vi "Ramsete_Execute_Ext_Odom.vi"(4 "Enabled":bool=TRUE, 6 "Reset":bool, 7 "RAMSETE_EXE_TUNING SI":T4={"B"=2.0, "Zeta"=0.7, "X Tolerance M"=2.0, "Y Tolerance M"=0.7, "Heading Tolerance RAD"=0.7, "Track Width M"=2.0, "Max Speed M/S"=2.0} {"Max Speed M/S" format="%13.4f"; "Track Width M" format="%13.4f"; "Heading Tolerance RAD" format="%13.4f"; "Y Tolerance M" format="%13.4f"; "X Tolerance M" format="%13.4f"; "Zeta" format="%13.4f"; "B" format="%13.4f"}, 9 "Current Pose SI":T1 {"ROTATION"."SIN" format="%13.4f"; "ROTATION"."COS" format="%13.4f"; "ROTATION"."VALUE" format="%13.4f"; "TRANSLATION"."Y" format="%14.3f"; "TRANSLATION"."X" format="%14.3f"}, 11 "TRAJ_STATE SI":T6 {"POSE"."ROTATION"."SIN" format="%13.4f"; "POSE"."ROTATION"."COS" format="%13.4f"; "POSE"."ROTATION"."VALUE" format="%13.4f"; "POSE"."TRANSLATION"."Y" format="%14.3f"; "POSE"."TRANSLATION"."X" format="%14.3f"}) -> (1 "AtReference":bool, 2 "Right Speed Dmd M/S":dbl, 3 "Left Speed Dmd M/S":dbl, 5 "outRAMSETE":T5={"B"=2.0, "Zeta"=0.7, "poseTolerance"={"TRANSLATION"={"X"=0.0, "Y"=0.0}, "ROTATION"={"VALUE"=0.0, "COS"=1.0, "SIN"=0.0}}, "poseError"={"TRANSLATION"={"X"=0.0, "Y"=0.0}, "ROTATION"={"VALUE"=0.0, "COS"=1.0, "SIN"=0.0}}, "Enabled"=TRUE} {"poseError"."ROTATION"."SIN" format="%13.4f"; "poseError"."ROTATION"."COS" format="%13.4f"; "poseError"."ROTATION"."VALUE" format="%13.4f"; "poseError"."TRANSLATION"."Y" format="%14.3f"; "poseError"."TRANSLATION"."X" format="%14.3f"; "poseTolerance"."ROTATION"."SIN" format="%13.4f"; "poseTolerance"."ROTATION"."COS" format="%13.4f"; "poseTolerance"."ROTATION"."VALUE" format="%13.4f"; "poseTolerance"."TRANSLATION"."Y" format="%14.3f"; "poseTolerance"."TRANSLATION"."X" format="%14.3f"; "Zeta" format="%12.3f"; "B" format="%12.3f"})   [LabVIEW 2019, in "Trajectory_Library.lvlib"]
doc: "Convienience function to create and calculate the ramsete control, returning normalized desired left and right speed setpoints \n\n\nParameters: \n - Ramsete EXE Tuning -- Packed data cluster containing the ramsete tuning parameters and Differntial Drive kinematics information. (SI Units)\n - TrajState - Desired trajectory state (SI Units)\n - Current Pose -- Current Pose2d robot location. (SI Units)\n - Reset -- Resets the Ramsete data structure.\n - Enabled -- When enabled uses the ramsete closed loop control to drive the left and right speed demand outputs. When disabled the trajectory data is directly converted to left and right speed demands.\n\n\nReturns:\n - Left Speed Dmd -- Left Speed demand (Meters/Second)\n - Right Speed Dmd -- Right Speed demand (Meters/Second)\n - Out Ramsete -- Updated Ramsete data structure (SI Units)\n - At Reference -- Set to TRUE when the current robot pose is withing the specified tolerance of the desired POSE from the trajectory state input."
uses:
  Trajectory_Library.lvlib
  TypeDef/TRAJ_STATE.ctl
  TypeDef/POSE2D.ctl
  TypeDef/TRANSLATION2D.ctl
  TypeDef/ROTATION2D.ctl
  TypeDef/RAMSETE.ctl
  TypeDef/RAMSETE_EXE_TUNING.ctl
  Rotation2d_CreateAngle.vi
  Translation2d_Create.vi
  <vilib>/Rock Robotics/SystemInterfaces/NetworkCommunication/NetComm_UsageReport_report.vi
  Globals/Util_LibraryGlobals.vi
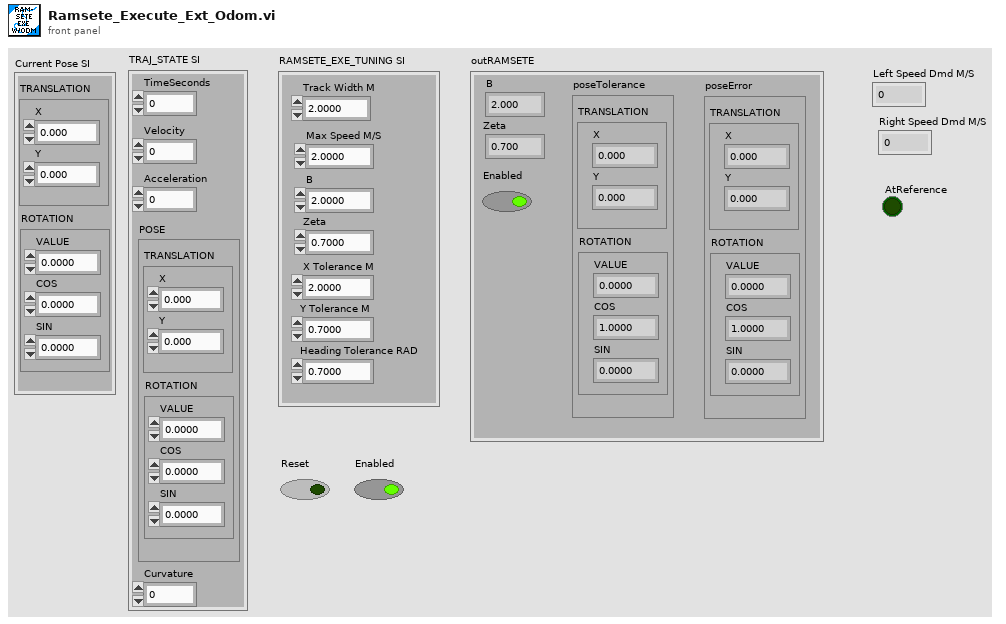
[diagram p1: front panel]
types:
  T1 = typedef "Trajectory_Library.lvlib/POSE2D.ctl" = cluster{"TRANSLATION":T2, "ROTATION":T3}
  T2 = typedef "Trajectory_Library.lvlib/TRANSLATION2D.ctl" = cluster{"X":dbl, "Y":dbl}
  T3 = typedef "Trajectory_Library.lvlib/ROTATION2D.ctl" = cluster{"VALUE":dbl, "COS":dbl, "SIN":dbl}
  T4 = typedef "Trajectory_Library.lvlib/RAMSETE_EXE_TUNING.ctl" = cluster{"B":dbl, "Zeta":dbl, "X Tolerance M":dbl, "Y Tolerance M":dbl, "Heading Tolerance RAD":dbl, "Track Width M":dbl, "Max Speed M/S":dbl}
  T5 = typedef "Trajectory_Library.lvlib/RAMSETE.ctl" = cluster{"B":dbl, "Zeta":dbl, "poseTolerance":T1, "poseError":T1, "Enabled":bool}
  T6 = typedef "Trajectory_Library.lvlib/TRAJ_STATE.ctl" = cluster{"TimeSeconds":dbl, "Velocity":dbl, "Acceleration":dbl, "POSE":T1, "Curvature":dbl}
  T7 = typedef "Trajectory_Library.lvlib/DIFF_DRIVE_KINEMATICS.ctl" = cluster{"TrackWidth_Meters":dbl}
  T8 = typedef "Trajectory_Library.lvlib/CHASSIS_SPEEDS.ctl" = cluster{"vX":dbl, "vY":dbl, "vOmega":dbl}
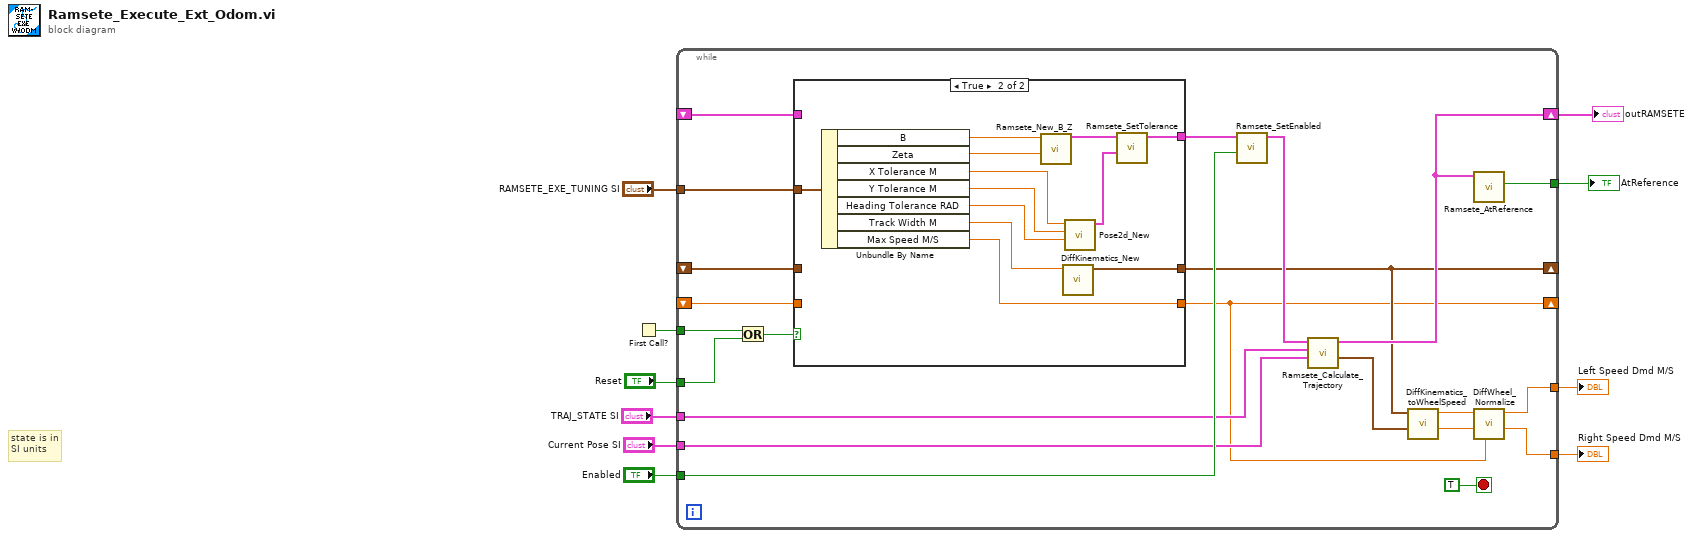
[diagram p0: block diagram]
diagram:
  # "state is in\nSI units"
  n1 = First Call?() -> (First Call?: T/F=w2:bool)
  n2 = while {
    tunnel: "RAMSETE_EXE_TUNING SI" -> [w13]
    tunnel: "TRAJ_STATE SI" -> [w17]
    tunnel: [w30] -> w6
    tunnel: [w29] -> w5
    tunnel: "Enabled" -> [w27]
    tunnel: "Reset" -> [w32]
    tunnel: [w21] -> w4
    tunnel: w2 -> [w26]
    shift-right: [w20] -> w8
    shift-left: _ -> [w25]
    tunnel: "Current Pose SI" -> [w16]
    shift-right: [w15] -> _
    shift-left: _ -> [w14]
    shift-right: [w12] -> _
    shift-left: _ -> [w11]
    stop <- TRUE stop-if-true
    n3 = Or(x=w26, y=w32) -> (x .or. y?=w31:bool)
    n4 = case shown="True" w31 {
      tunnel: [w35 w45] -> w28
      tunnel: w25 -> [w35 _]
      tunnel: [w34 w44] -> w15
      tunnel: w14 -> [w34 _]
      tunnel: [w33 w36] -> w12
      tunnel: w13 -> [_ w43]
      tunnel: w11 -> [w33 _]
      frame False {
      }
      frame True {
        n5 = Unbundle By Name(w43) -> ("B"=w42:dbl, "Zeta"=w41:dbl, "X Tolerance M"=w40:dbl, "Y Tolerance M"=w39:dbl, "Heading Tolerance RAD"=w38:dbl, "Track Width M"=w37:dbl, "Max Speed M/S"=w36:dbl)
        n6 = call "Ramsete_New_B_Z.vi"("Zeta"=w41, "B"=w42) -> ("outRAMSETE"=w47:T5)  [unwired: 9 in]
        n7 = call "DiffKinematics_New.vi"("TrackWidth_Meters"=w37) -> ("DIFF_DRIVE_KINEMATICS"=w44:T7)  [unwired: 10 in]
        n8 = call "Pose2d_New.vi"("Heading"=w38, "Y"=w39, "X"=w40) -> ("out POSe"=w46:T1)  [unwired: 8 in]
        n9 = call "Ramsete_SetTolerance.vi"("tolerancePose"=w46, "inRAMSETE"=w47) -> ("outRAMSETE"=w45:T5)  [unwired: 9 in]
      }
    }
    n10 = call "Ramsete_SetEnabled.vi"("Enabled"=w27, "inRAMSETE"=w28) -> ("outRAMSETE"=w22:T5)  [unwired: 9 in]
    n11 = call "Ramsete_Calculate_Trajectory.vi"("CurrentPOSE"=w16, "TRAJ_STATE"=w17, "inRAMSETE"=w22) -> ("CHASSIS Speeds"=w23:T8, "outRAMSETE"=w20:T5)  [unwired: 7 in]
    n12 = call "DiffKinematics_toWheelSpeed.vi"("CHASSIS Speed"=w23, "DIFF_DRIVE_KINEMATICS"=w15) -> ("RightVelocity"=w18:dbl, "LeftVelocity"=w19:dbl)  [unwired: 8 in]
    n13 = call "Ramsete_AtReference.vi"("RAMSETE"=w20) -> ("AtReference"=w21:bool)  [unwired: 10 in]
    n14 = call "DiffWheel_Normalize.vi"("Max Speed"=w12, "Right Wheel Demand"=w18, "Left Wheel Demand"=w19) -> ("Normalized Right Wheel Demand"=w29:dbl, "Normalized Left Wheel Demand"=w30:dbl)  [unwired: 7 in]
  }
  "outRAMSETE" <- w8
  "Left Speed Dmd M/S" <- w6
  "Right Speed Dmd M/S" <- w5
  "AtReference" <- w4
